vi "TriangleContinuityTest.vi"(7 "Pulse Positions Array":T1[](array[typedef]), 9 "Acq Block Number":i32, 10 "Waveforms":waveform(sgl)[](array[waveform]), 11 "Qbus in":refnum<class "Qbus.lvclass">) -> ()   [LabVIEW 2017]
uses:
  <vilib>/addons/Qbus/Qbus.lvclass
  <vilib>/addons/InsightCM/Utilities/Analysis/Shared/controls/PulsePositions.ctl
  <vilib>/addons/InsightCM/Utilities/Analysis/Shared/AnalysisHelper.lvlib
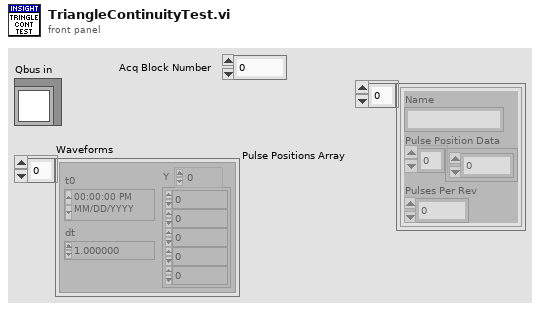
[diagram p1: front panel]
types:
  T1 = typedef "AnalysisHelper.lvlib/PulsePositions.ctl" = cluster{"Name":string, "Pulse Position Data":dbl[], "Pulses Per Rev":i32}
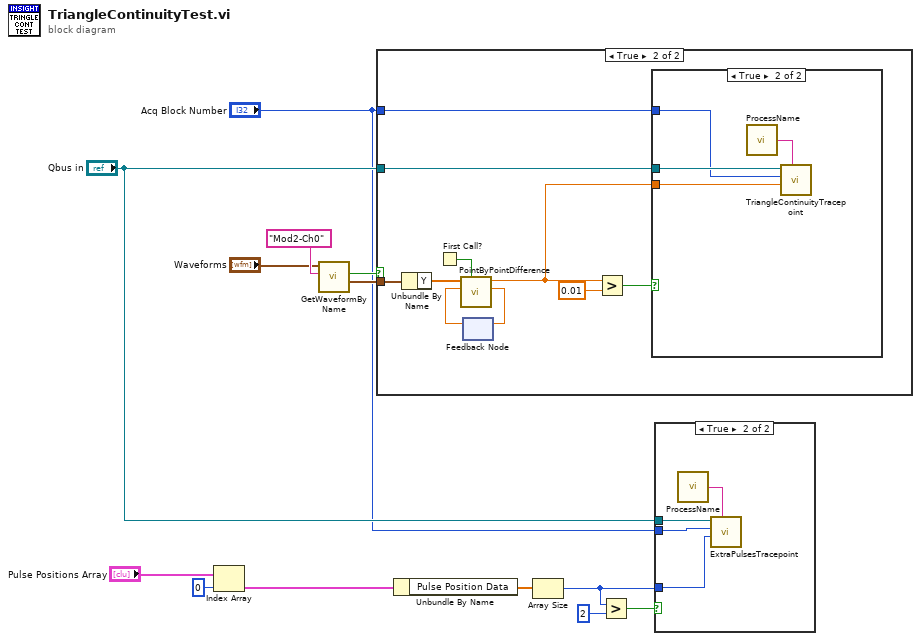
[diagram p0: block diagram]
diagram:
  n1 = Index Array(array="Pulse Positions Array", index=0) -> (element=w7:T1)
  n2 = call <vilib>:"GetWaveformByName.vi"("Channel Name"="Mod2-Ch0", "Acq Waveforms"="Waveforms") -> ("Waveform"=w12:waveform(sgl), "Found?"=w11:bool)  [unwired: 6 in, 2 out]
  n3 = case shown="True" w11 {
    tunnel: "Qbus in" -> [_ w23]
    tunnel: w12 -> [_ w21]
    tunnel: "Acq Block Number" -> [_ w16]
    frame False {
    }
    frame True {
      n4 = Unbundle By Name(w21) -> ("Y"=w22:sgl[])
      n5 = First Call?() -> (First Call?: T/F=w15:bool)
      n6 = feedback #1() -> (w19:dbl)  [unwired: 1 in]
      n7 = call <vilib>:"PointByPointDifference.vi"("reset?"=w15, "initial condition"=w19, "array"=w22) -> ("last point"=w20:dbl, "max difference"=w14:dbl)  [unwired: 6 in, 1 out]
      n8 = feedback-in #1(w20) -> ()
      n9 = Greater?(x=w14, y=0.01) -> (0:w17:bool)
      n10 = case shown="True" w17 {
        tunnel: w23 -> [_ w27]
        tunnel: w16 -> [_ w25]
        tunnel: w14 -> [_ w24]
        frame False {
        }
        frame True {
          n11 = call <vilib>:"ProcessName.vi"() -> ("process name"=w26:string)  [unwired: 5 in]
          n12 = call <vilib>:"TriangleContinuityTracepoint.vi"("service name"=w26, "max difference"=w24, "Acq Block Number"=w25, "Qbus in"=w27) -> ()  [unwired: 7 in, 1 out]
        }
      }
    }
  }
  n13 = Unbundle By Name(w7) -> ("Pulse Position Data"=w6:dbl[])
  n14 = Array Size(array=w6) -> (size(s)=w1:i32)
  n15 = Greater?(x=w1, y=2) -> (0:w5:bool)
  n16 = case shown="True" w5 {
    tunnel: "Qbus in" -> [_ w31]
    tunnel: "Acq Block Number" -> [_ w29]
    tunnel: w1 -> [_ w28]
    frame False {
    }
    frame True {
      n17 = call <vilib>:"ProcessName.vi"() -> ("process name"=w30:string)  [unwired: 5 in]
      n18 = call <vilib>:"ExtraPulsesTracepoint.vi"("service name"=w30, "pulses"=w28, "Acq Block Number"=w29, "Qbus in"=w31) -> ()  [unwired: 7 in, 1 out]
    }
  }
